vi "Generic Camera Wait For New Frame.vi"(0 "Camera Notifier Name":string, 13 "Wait No. (1)":u32=1) -> (4 "Camera Notifier Name (Dup)":string, 15 "Image Ref":T1)   [LabVIEW 2025]
uses:
  <vilib>/vision/Image Controls.llb/IMAQ Image.ctl
  Camera Controls/Generic Camera Actions.ctl
  Camera Controls/Camera IMAQ Key Info.ctl
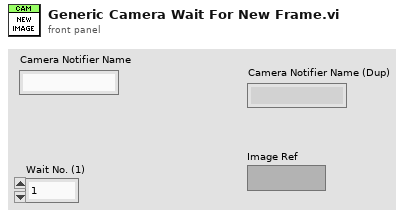
[diagram p1: front panel]
types:
  T1 = typedef "IMAQ Image.ctl" = refnum<image>
  T2 = typedef "Generic Camera Actions.ctl" = enum16{"Status", "Live Preview", "Capture", "Abort", "Set Exposure Time (s)", "Get Exposure Time (s)", "Record Settings", "Binning", "Set ROI", "Get ROI", "Defect Correction On?", "Cooler On?", "Fan On?", "Quit"}
  T3 = typedef "Camera IMAQ Key Info.ctl" = cluster{"Frame":u32, "Sensor Height":i32, "Sensor Width":i32, "ROI Height":i32, "ROI Width":i32, "ROI Enable?":bool, "Bit per Pixel":u8}
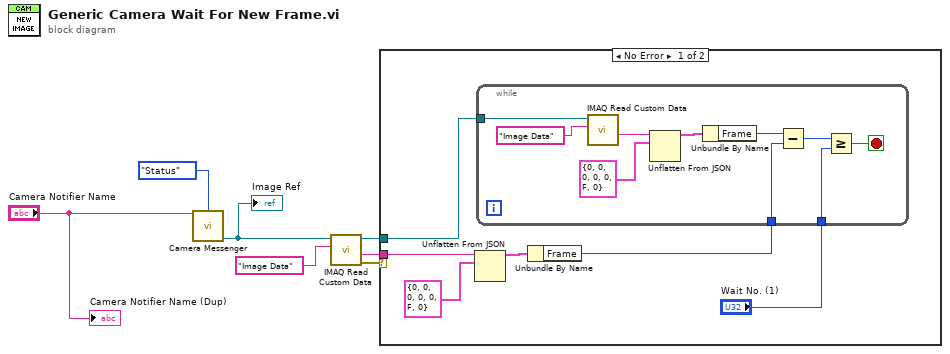
[diagram p0: block diagram]
diagram:
  n1 = call "Camera Messenger.vi"("Notifier Name"="Camera Notifier Name", "General Camera Actions"=Generic_Camera_Actions."Status") -> ("Image Ref"=w2:T1)  [unwired: 8 in, 5 out]
  "Image Ref" <- w2
  n2 = call "IMAQ Read Custom Data"("Key"="Image Data", "Image"=w2) -> ("error out"=w1:errorcluster, "Custom Data Out"=w7:string, "Image (duplicate)"=w5:T1)  [unwired: 7 in]
  n3 = case shown="No Error" w1 {
    tunnel: w7 -> [w11 _]
    tunnel: w5 -> [w10 _]
    frame No Error {
      n4 = Unflatten From JSON(JSON string=w11, type and defaults=T3 {"Frame"=0, "Sensor Height"=0, "Sensor Width"=0, "ROI Height"=0, "ROI Width"=0, "ROI Enable?"=FALSE, "Bit per Pixel"=0} ("Camera IMAQ Key Info")) -> (value=w13:T3)  [unwired: 5 in, 1 out]
      n5 = Unbundle By Name(w13) -> ("Frame"=w9:u32)
      n6 = while {
        tunnel: w10 -> [w19]
        tunnel: w9 -> [w17]
        tunnel: "Wait No. (1)" -> [w14]
        stop <- w15 stop-if-true
        n7 = call "IMAQ Read Custom Data"("Key"="Image Data", "Image"=w19) -> ("Custom Data Out"=w21:string)  [unwired: 7 in, 2 out]
        n8 = Unflatten From JSON(JSON string=w21, type and defaults=T3 {"Frame"=0, "Sensor Height"=0, "Sensor Width"=0, "ROI Height"=0, "ROI Width"=0, "ROI Enable?"=FALSE, "Bit per Pixel"=0} ("Camera IMAQ Key Info")) -> (value=w23:T3)  [unwired: 5 in, 1 out]
        n9 = Unbundle By Name(w23) -> ("Frame"=w18:u32)
        n10 = Subtract(x=w18, y=w17) -> (x-y=w16:u32)
        n11 = Greater Or Equal?(x=w16, y=w14) -> (x >= y?=w15:bool)
      }
    }
    frame Error {
    }
  }
  "Camera Notifier Name (Dup)" <- "Camera Notifier Name"
